vi "BuildCustomDashBoardData.vi"   [LabVIEW 2014]
doc: "This VI builds data and sends it back to the dashboard PC program. By default it sends back the raw values for the first analog, digital, and solenoid module. Modify it to send back the data you want to view. Consider adding higher level data to the Dashboard Datatype.ctl and to this VI. Then update the Dashboard to display the data however you like.\n\nThis software is licensed. Open the labview\\readme\\WPI Robotics Library Open Source License.txt file for more information."
uses:
  typedefs/test/test controls.ctl
  typedefs/fg_getset.ctl
  typedefs/dashboard/DashboardEnable.ctl
  <vilib>/Rock Robotics/SystemInterfaces/Typedef/FPGA_TypedefDigitalModule.ctl
  typedefs/dashboard/misc dash data.ctl
  <vilib>/Rock Robotics/WPI/Solenoid/WPI_SolenoidDevRef.ctl
  <vilib>/Rock Robotics/WPI/Solenoid/WPI_SolenoidChannel.ctl
  <vilib>/Rock Robotics/WPI/AnalogModule/WPI_AnalogModuleDevStatus.ctl
  <vilib>/Rock Robotics/SystemInterfaces/Typedef/FPGA_TypedefAnalogModule.ctl
  <vilib>/Rock Robotics/SystemInterfaces/AI/FPGA_AIChannel.ctl
  <vilib>/Rock Robotics/WPI/DriverStation/WPI_DriverStationDigitalData.ctl
  <vilib>/Rock Robotics/SystemInterfaces/DIO/FPGA_DIOPWMChannel.ctl
  <vilib>/Rock Robotics/WPI/Compressor/WPI_CompressorGetSetRefNum.vi
  <vilib>/Rock Robotics/Network Tables/SD Write Numeric Array.vi
  <vilib>/Rock Robotics/SystemInterfaces/System/FPGA_SystemGet.vi
  <vilib>/Rock Robotics/WPI/Solenoid/Deprecated/WPI_SolenoidGetBool.vi
  <vilib>/Rock Robotics/Network Tables/SD Write Boolean Array.vi
  <vilib>/NI_Real-Time Target Support.lvlib
panel:
  # "Generate Dashboard Data and Send it"
  # "Note: Test code calls some dashboard data, which is gotten there not here"
types:
  T1 = typedef "WPI_AnalogModuleDevStatus.ctl" = cluster{"DevStatus":errorcluster, "Controller":T2}
  T2 = typedef "FPGA_TypedefAnalogModule.ctl" = enum16{"Controller 1"}
  T3 = typedef "FPGA_AIChannel.ctl" = enum8{"AI 0", "AI 1", "AI 2", "AI 3", "AI MXP 0", "AI MXP 1", "AI MXP 2", "AI MXP 3", "Invalid"}
  T4 = typedef "FPGA_TypedefDigitalModule.ctl" = enum16{"Controller 1"}
  T5 = typedef "WPI_DriverStationDigitalData.ctl" = cluster{"Relay Fwd":u8, "Relay Rev":u8, "GPIO":u16, "GPIO_OE":u16, "PWM":cluster{"PWM[0]":u8, "PWM[1]":u8, "PWM[2]":u8, "PWM[3]":u8, "PWM[4]":u8, "PWM[5]":u8, "PWM[6]":u8, "PWM[7]":u8, "PWM[8]":u8, "PWM[9]":u8}}
  T6 = typedef "FPGA_DIOPWMChannel.ctl" = enum8{"PWM 0", "PWM 1", "PWM 2", "PWM 3", "PWM 4", "PWM 5", "PWM 6", "PWM 7", "PWM 8", "PWM 9", "PWM MXP 0", "PWM MXP 1", "PWM MXP 2", "PWM MXP 3", "PWM MXP 4", "PWM MXP 5", "PWM MXP 6", "PWM MXP 7", "PWM MXP 8", "PWM MXP 9", "Invalid"}
  T7 = typedef "WPI_SolenoidChannel.ctl" = enum8{"Solenoid 0", "Solenoid 1", "Solenoid 2", "Solenoid 3", "Solenoid 4", "Solenoid 5", "Solenoid 6", "Solenoid 7", "Invalid"}
  T8 = typedef "WPI_SolenoidDevRef.ctl" = cluster{"DevStatus":errorcluster, "Pneumatics Control Module":u8, "Forward Solenoid Channel":T7, "Reverse Solenoid Channel":T7}
  T9 = typedef "misc dash data.ctl" = cluster{"Total (%)":dbl, "Vision mSPI":u32, "Main mSPI":u32, "Vision":cluster{"distance":dbl}, "Enabled?":bool}
  T10 = typedef "DashboardEnable.ctl" = cluster{"Analog I/O":bool[], "Digital I/O":bool, "Solenoids":bool}
  T11 = typedef "subStates.ctl" = enum16{"null", "wait", "driver control", "auto", "manual override", "hold position", "rotate", "test", "end"}
  T12 = typedef "FPGA_DIODevRef.ctl" = cluster{"DevStatus":errorcluster, "Controller":T4}
  T13 = cluster{"[0]":u16, "[1]":u16, "[2]":u16, "[3]":u16, "[4]":u16, "[5]":u16, "[6]":u16, "[7]":u16, "[8]":u16, "[9]":u16}
  T14 = typedef "WPI_EncoderDevRef.ctl" = cluster{"DevStatus":errorcluster, "EncoderIndex":T15, "CounterIndex":T16, "DistancePerCount":dbl, "Decoding Type":T17}
  T15 = typedef "FPGA_EncoderIdx.ctl" = enum8{"Enc 0", "Enc 1", "Enc 2", "Enc 3", "Enc 4", "Enc 5", "Enc 6", "Enc 7", "Invalid"}
  T16 = typedef "FPGA_CounterCtrSystemIndex.ctl" = enum8{"Ctr 0", "Ctr 1", "Ctr 2", "Ctr 3", "Ctr 4", "Ctr 5", "Ctr 6", "Ctr 7", "Invalid"}
  T17 = typedef "WPI_EncoderType.ctl" = enum16{"1x", "2x", "4x"}
  T18 = typedef "WPI_CompressorDevRef.ctl" = cluster{"DevStatus":errorcluster, "Pneumatics Control Module":u8}
  T19 = typedef "fg_getset.ctl" = enum16{"Get", "Set"}
  T20 = typedef "NI_Real-Time Target Support.lvlib/RT CPU Load.ctl" = cluster{"Total (%)":dbl, "Time Critical (%)":dbl, "Timed Structures (%)":dbl, "High (%)":dbl, "Above Normal (%)":dbl, "Normal (%)":dbl, "Background (%)":dbl, "Idle (%)":dbl, "ISR (%)":dbl}
  T21 = cluster{"Vision mSPI":u32, "Main mSPI":u32, "Dash mSPI":u32}
  T22 = typedef "test controls.ctl" = cluster{"Button":bool, "Switch":bool, "Slider":dbl}
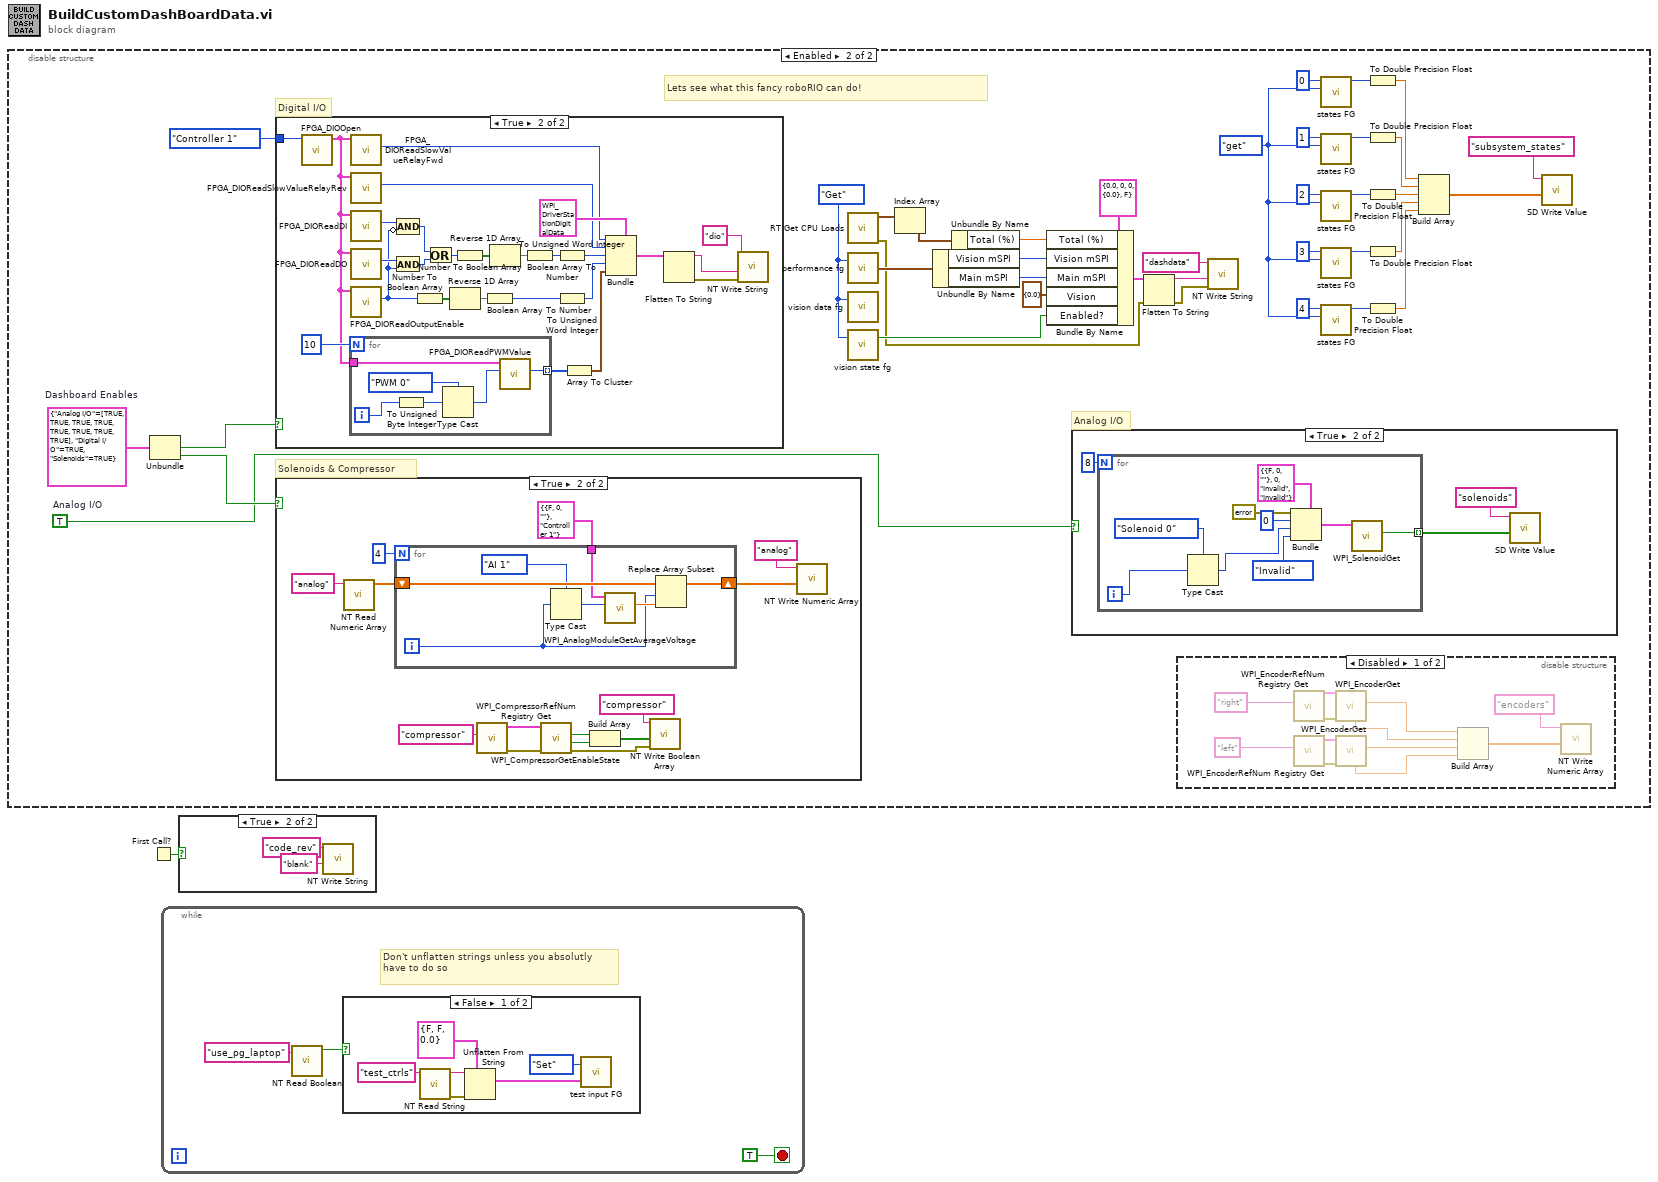
[diagram p0: block diagram]
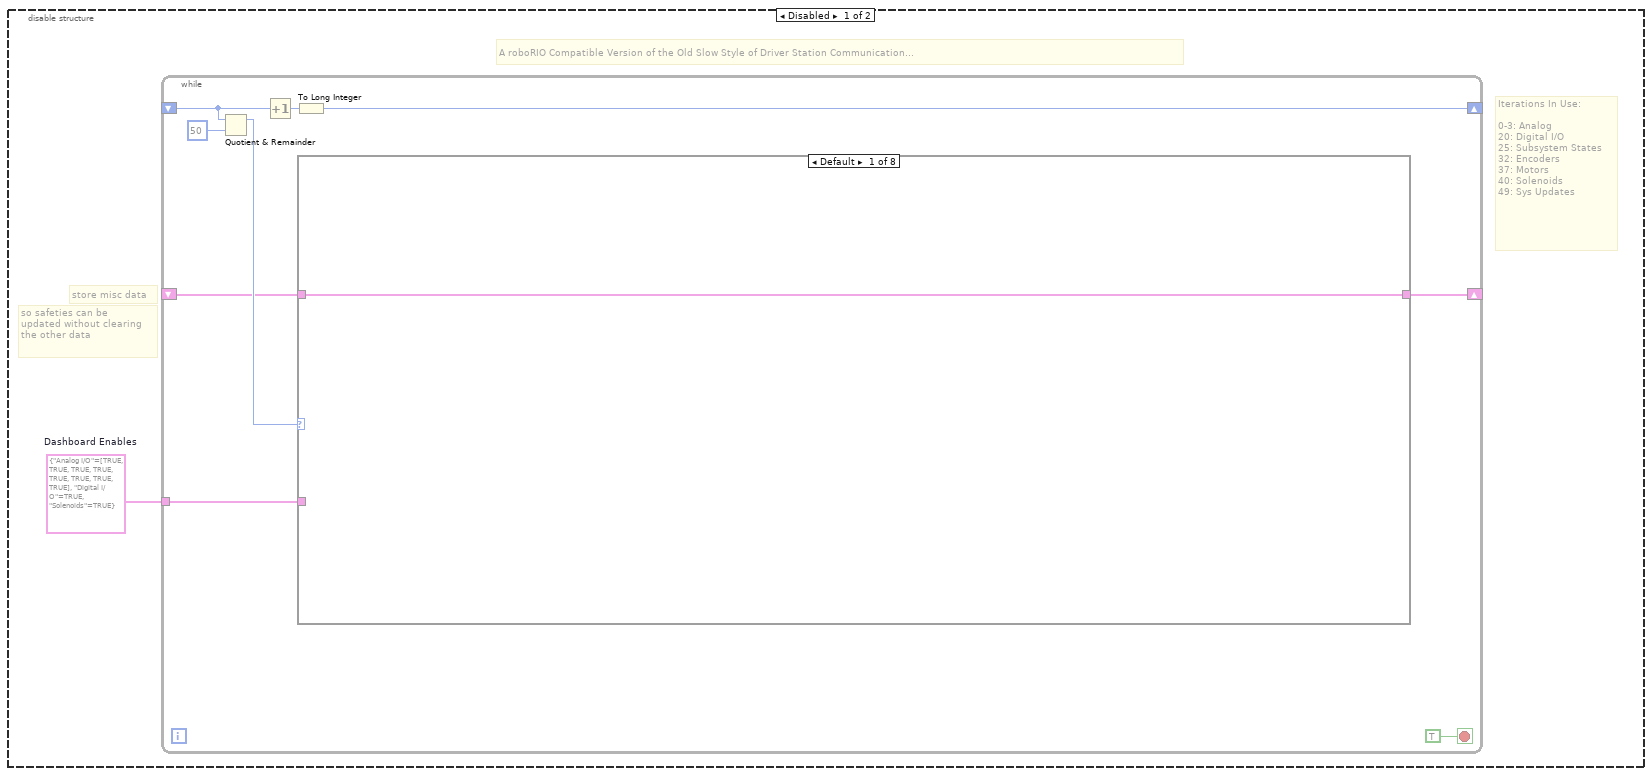
[diagram p2: hidden frame]
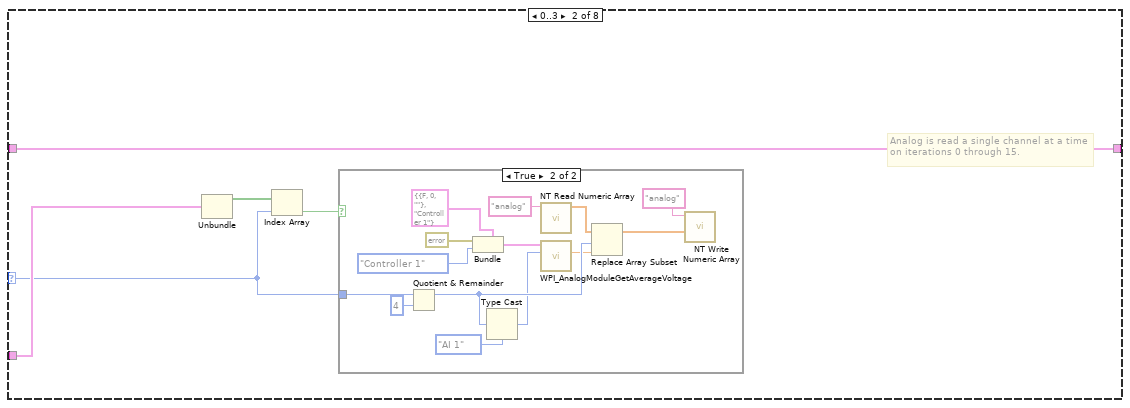
[diagram p3: hidden frame]
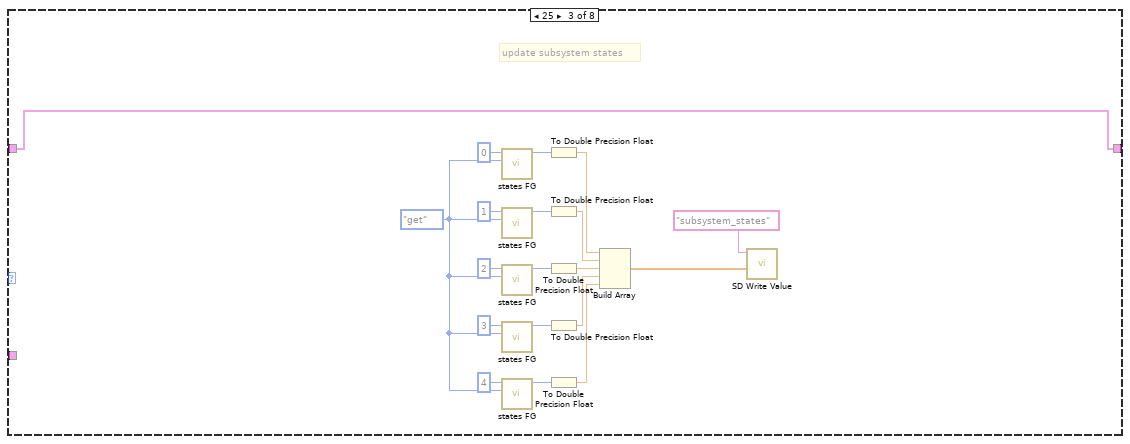
[diagram p5: hidden frame]
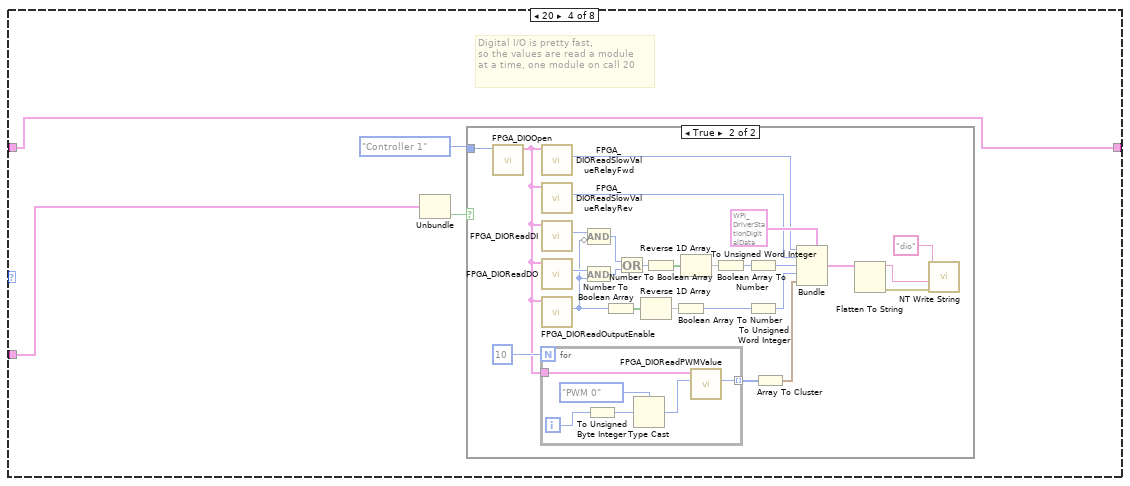
[diagram p6: hidden frame]
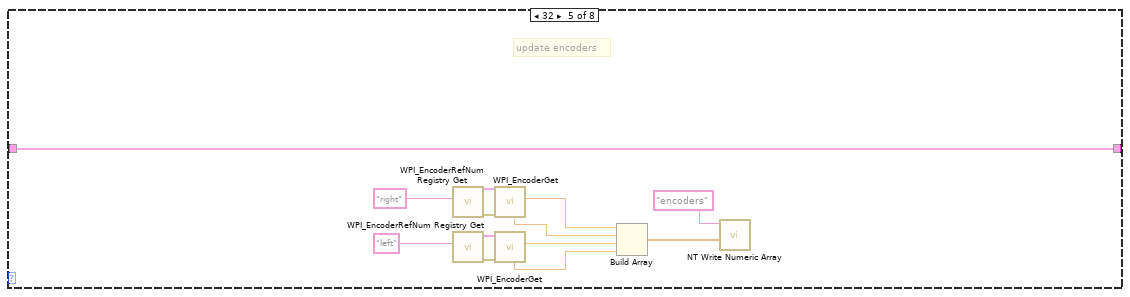
[diagram p8: hidden frame]
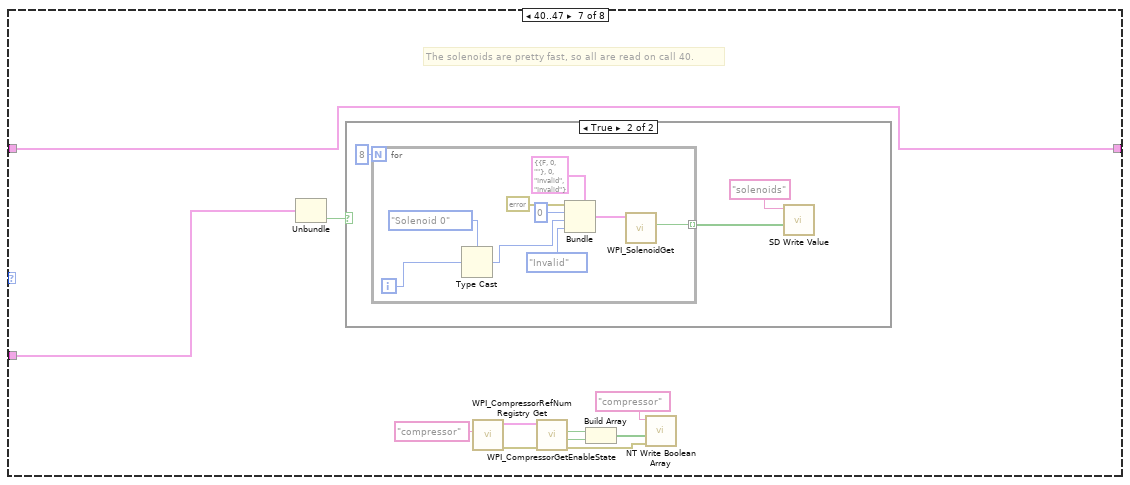
[diagram p10: hidden frame]
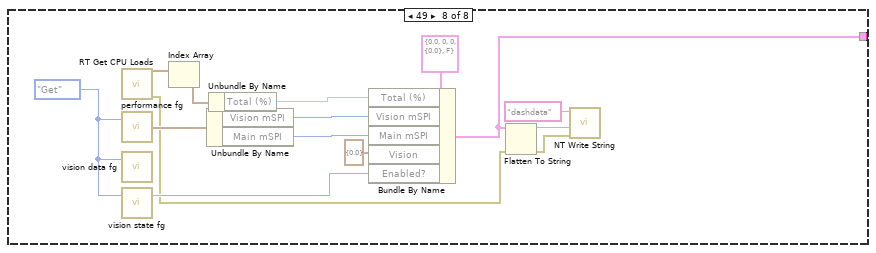
[diagram p12: hidden frame]
diagram:
  n1 = disable-structure shown="Enabled" {
    frame Disabled {
      w2 = T10 {"Analog I/O"=[TRUE, TRUE, TRUE, TRUE, TRUE, TRUE, TRUE, TRUE], "Digital I/O"=TRUE, "Solenoids"=TRUE}  # Dashboard Enables
      # "A roboRIO Compatible Version of the Old Slow Style of Driver Station Communication..."
      # "so safeties can be\nupdated without clearing\nthe other data"
      # "store misc data"
      # "Iterations In Use:\n\n0-3: Analog\n20: Digital I/O \n25: Subsystem States\n32: Encoders\n37: Motors\n40: Solenoids\n49: Sys Updates"
      n2 = while {
        shift-right: [w8] -> _
        shift-left: _ -> [w9]
        tunnel: w2 -> [w6]
        shift-right: [w4] -> _
        shift-left: _ -> [w3]
        stop <- TRUE stop-if-true
        n3 = Quotient & Remainder(x=w9, y=50) -> (x-y*floor(x/y)=w5:i32)  [unwired: 1 out]
        n4 = Increment(x=w9) -> (x+1=w10:i32)
        n5 = To Long Integer(number=w10) -> (32bit integer=w8:i32)
        n6 = case shown="Default" w5 {
          selector: w5 -> [_ w16 _ _ _ _ _ _]
          tunnel: w6 -> [_ w17 _ w54 _ _ w111 _]
          tunnel: [w12 w14 w33 w51 w89 w100 w102 w125] -> w4
          tunnel: w3 -> [w12 w14 w33 w51 w89 w100 w102 _]
          frame Default {
          }
          frame 0..3 {
            # "Analog is read a single channel at a time\non iterations 0 through 15."
            n7 = Unbundle(w17) -> ("Analog I/O"=w13:bool[])  [unwired: 2 out]
            n8 = Index Array(array=w13, index=w16) -> (element=w15:bool)
            n9 = case shown="True" w15 {
              tunnel: w16 -> [_ w29]
              frame False {
              }
              frame True {
                n10 = Quotient & Remainder(x=w29, y=4) -> (x-y*floor(x/y)=w23:i32)  [unwired: 1 out]
                n11 = Bundle(cluster=T1 {"DevStatus"={"status"=FALSE, "code"=0, "source"=""}, "Controller"=enum."Controller 1"} ("AnalogModuleDevStatus"), "DevStatus"=errorcluster {"status"=FALSE, "code"=0, "source"=""}, "Controller"=FPGA_TypedefAnalogModule."Controller 1") -> (w20:T1)
                n12 = Type Cast(type=FPGA_AIChannel."AI 1" ("Channel"), x=w23) -> (*(type *) &x=w22:T3)
                n13 = call <vilib>:"NT Read Numeric Array.vi"("Name"="analog") -> ("Numeric Array"=w27:dbl[])  [unwired: 9 in, 1 out]
                n14 = call <vilib>:"WPI_AnalogModuleGetAverageVoltage.vi"("Channel"=w22, "AnalogModuleDevStatus"=w20) -> ("Average Voltage"=w18:dbl)  [unwired: 1 in, 8 out]
                n15 = Replace Array Subset(array=w27, new element=w18, index=w23) -> (w25:dbl[])
                n16 = call <vilib>:"NT Write Numeric Array.vi"("Numeric Array"=w25, "Name"="analog") -> ()  [unwired: 9 in, 1 out]
              }
            }
          }
          frame 25 {
            w45 = enum16{"set", "get"}."get" ("menu (get)")
            # "update subsystem states"
            n17 = call "states FG.vi"("menu (get)"=w45, "Loop ID"=0) -> ("subState out"=w42:T11)  [unwired: 6 in, 3 out]
            n18 = call "states FG.vi"("menu (get)"=w45, "Loop ID"=1) -> ("subState out"=w43:T11)  [unwired: 6 in, 3 out]
            n19 = call "states FG.vi"("menu (get)"=w45, "Loop ID"=2) -> ("subState out"=w44:T11)  [unwired: 6 in, 3 out]
            n20 = call "states FG.vi"("menu (get)"=w45, "Loop ID"=3) -> ("subState out"=w41:T11)  [unwired: 6 in, 3 out]
            n21 = call "states FG.vi"("menu (get)"=w45, "Loop ID"=4) -> ("subState out"=w40:T11)  [unwired: 6 in, 3 out]
            n22 = To Double Precision Float(number=w42) -> (double precision float=w38:dbl)
            n23 = To Double Precision Float(number=w43) -> (double precision float=w37:dbl)
            n24 = To Double Precision Float(number=w44) -> (double precision float=w36:dbl)
            n25 = To Double Precision Float(number=w41) -> (double precision float=w35:dbl)
            n26 = To Double Precision Float(number=w40) -> (double precision float=w34:dbl)
            n27 = Build Array(w38, w37, w36, w35, w34) -> (w32:dbl[])
            n28 = call-poly <vilib>:"SD Write Value.vi"("Numeric Array"=w32, "Name"="subsystem_states") -> ()  [unwired: 8 in, 2 out]
          }
          frame 20 {
            # "Digital I/O is pretty fast,\nso the values are read a module\nat a time, one module on call 20"
            n29 = Unbundle(w54) -> ("Solenoids"=w52:bool)  [unwired: 2 out]
            n30 = case shown="True" w52 {
              tunnel: FPGA_TypedefDigitalModule."Controller 1" ("Module (Module 1)") -> [_ w61]
              frame False {
              }
              frame True {
                n31 = call <vilib>:"FPGA_DIOOpen.vi"("Controller"=w61) -> ("DIODeviceRef"=w77:T12)  [unwired: 1 in, 9 out]
                n32 = for {
                  N: 10 -> [_]
                  tunnel: w77 -> [w86]
                  tunnel: [w84] -> w78 mode=indexing
                  i -> [w85]
                  n33 = To Unsigned Byte Integer(number=w85) -> (unsigned 8bit integer=w83:u8)
                  n34 = Type Cast(type=FPGA_DIOPWMChannel."PWM 0" ("PWMChannel"), x=w83) -> (*(type *) &x=w81:T6)
                  n35 = call <vilib>:"FPGA_DIOReadPWMValue.vi"("PWMChannel"=w81, "DIODeviceRef In"=w86) -> ("PWMValue"=w84:u16)  [unwired: 1 in, 8 out]
                }
                n36 = call <vilib>:"FPGA_DIOReadSlowValueRelayFwd.vi"("DIODeviceRef In"=w77) -> ("Relay Forward"=w70:u8)  [unwired: 1 in, 9 out]
                n37 = call <vilib>:"FPGA_DIOReadSlowValueRelayRev.vi"("DIODeviceRef In"=w77) -> ("Relay Reverse"=w71:u8)  [unwired: 1 in, 9 out]
                n38 = call <vilib>:"FPGA_DIOReadDI.vi"("DIODeviceRef In"=w77) -> ("DI"=w75:u32)  [unwired: 1 in, 9 out]
                n39 = call <vilib>:"FPGA_DIOReadDO.vi"("DIODeviceRef In"=w77) -> ("DO"=w74:u32)  [unwired: 1 in, 9 out]
                n40 = call <vilib>:"FPGA_DIOReadOutputEnable.vi"("DIODeviceRef In"=w77) -> ("OutputEnable"=w65:u32)  [unwired: 1 in, 9 out]
                n41 = And(x=w74, y=w65) -> (x .and. y?=w73:u32)
                n42 = Compound Arithmetic op=AND(w75, invert w65) -> (w72:u32)
                n43 = Number To Boolean Array(number=w65) -> (Boolean array=w67:bool[])
                n44 = Or(x=w72, y=w73) -> (x .or. y?=w63:u32)
                n45 = Reverse 1D Array(array=w67) -> (reversed array=w66:bool[])
                n46 = Number To Boolean Array(number=w63) -> (Boolean array=w68:bool[])
                n47 = Boolean Array To Number(Boolean array=w66) -> (number=w64:u32)
                n48 = Reverse 1D Array(array=w68) -> (reversed array=w69:bool[])
                n49 = Boolean Array To Number(Boolean array=w69) -> (number=w62:u32)
                n50 = To Unsigned Word Integer(number=w62) -> (unsigned 16bit integer=w55:u16)
                n51 = To Unsigned Word Integer(number=w64) -> (unsigned 16bit integer=w56:u16)
                n52 = Array To Cluster(array=w78) -> (cluster=w76:T13)
                n53 = Bundle(cluster=T5 {"Relay Fwd"=0, "Relay Rev"=0, "GPIO"=0, "GPIO_OE"=0, "PWM"={"PWM[0]"=0, "PWM[1]"=0, "PWM[2]"=0, "PWM[3]"=0, "PWM[4]"=0, "PWM[5]"=0, "PWM[6]"=0, "PWM[7]"=0, "PWM[8]"=0, "PWM[9]"=0}} ("DigitalModule"), "Relay Fwd"=w70, "Relay Rev"=w71, "GPIO"=w55, "GPIO_OE"=w56, "PWM"=w76) -> (w60:T5)
                n54 = Flatten To String(anything=w60) -> (data string=w58:string, error out=w59:errorcluster)  [unwired: 1 in, 3 out]
                n55 = call <vilib>:"NT Write String.vi"("error in"=w59, "String"=w58, "Name"="dio") -> ()  [unwired: 8 in, 1 out]
              }
            }
          }
          frame 32 {
            # "update encoders"
            n56 = call <vilib>:"WPI_EncoderRefNum Registry Get.vi"("refnum name"="right") -> ("error out"=w97:errorcluster, "EncoderDevRef"=w96:T14)  [unwired: 9 in]
            n57 = call <vilib>:"WPI_EncoderRefNum Registry Get.vi"("refnum name"="left") -> ("error out"=w94:errorcluster, "EncoderDevRef"=w95:T14)  [unwired: 9 in]
            n58 = call <vilib>:"WPI_EncoderGet.vi"("error in (no error)"=w97, "EncoderDevRef"=w96) -> ("Distance"=w93:dbl, "Rate"=w88:dbl)  [unwired: 4 in, 4 out]
            n59 = call <vilib>:"WPI_EncoderGet.vi"("error in (no error)"=w94, "EncoderDevRef"=w95) -> ("Distance"=w92:dbl, "Rate"=w91:dbl)  [unwired: 4 in, 4 out]
            n60 = Build Array(w93, w88, w92, w91) -> (w90:dbl[])
            n61 = call <vilib>:"NT Write Numeric Array.vi"("Numeric Array"=w90, "Name"="encoders") -> ()  [unwired: 9 in, 1 out]
          }
          frame 37 {
            # "update motor array"
          }
          frame 40..47 {
            # "The solenoids are pretty fast, so all are read on call 40."
            n62 = Unbundle(w111) -> ("Solenoids"=w101:bool)  [unwired: 2 out]
            n63 = case shown="True" w101 {
              frame False {
              }
              frame True {
                n64 = for {
                  N: 8 -> [_]
                  tunnel: [w115] -> w113 mode=indexing
                  i -> [w117]
                  n65 = Type Cast(type=WPI_SolenoidChannel."Solenoid 0" ("Forward Solenoid Channel"), x=w117) -> (*(type *) &x=w116:T7)
                  n66 = Bundle(cluster=T8 {"DevStatus"={"status"=FALSE, "code"=0, "source"=""}, "Pneumatics Control Module"=0, "Forward Solenoid Channel"=enum."Invalid", "Reverse Solenoid Channel"=enum."Invalid"} ("SolenoidDevRef"), "DevStatus"=errorcluster {"status"=FALSE, "code"=0, "source"=""}, "Pneumatics Control Module"=u8 0, "Forward Solenoid Channel"=w116, "Reverse Solenoid Channel"=WPI_SolenoidChannel."Invalid") -> (w122:T8)
                  n67 = call-poly <vilib>:"WPI_SolenoidGet.vi"("SolenoidDevRef"=w122) -> ("Value"=w115:bool)  [unwired: 8 in, 2 out]
                }
                n68 = call-poly <vilib>:"SD Write Value.vi"("Boolean Array"=w113, "Name"="solenoids") -> ()  [unwired: 8 in, 2 out]
              }
            }
            n69 = call <vilib>:"WPI_CompressorRefNum Registry Get.vi"("refnum name"="compressor") -> ("error out"=w107:errorcluster, "CompressorDevRef"=w108:T18)  [unwired: 9 in]
            n70 = call <vilib>:"WPI_CompressorGetEnableState.vi"("error in (no error)"=w107, "CompressorDevRef"=w108) -> ("error out"=w103:errorcluster, "Compressor Running"=w105:bool, "Enabled"=w106:bool)  [unwired: 6 in, 1 out]
            n71 = Build Array(w106, w105) -> (w104:bool[])
            n72 = call <vilib>:"NT Write Boolean Array.vi"("error in"=w103, "Boolean Array"=w104, "Name"="compressor") -> ()  [unwired: 8 in, 1 out]
          }
          frame 49 {
            w135 = fg_getset."Get" ("Menu")
            n73 = call <vilib>:"RT Get CPU Loads.vi"() -> ("error out"=w126:errorcluster, "CPU loads"=w137:T20[])  [unwired: 10 in]
            n74 = call "performance fg.vi"("Menu"=w135) -> ("Output"=w136:T21)  [unwired: 1 in]
            n75 = call "vision data fg.vi"("Menu"=w135) -> ()  [unwired: 1 in, 1 out]
            n76 = call "vision state fg.vi"("Menu"=w135) -> ("Enabled?"=w133:bool)  [unwired: 1 in, 1 out]
            n77 = Index Array(array=w137) -> (element=w138:T20)  [unwired: 1 in]
            n78 = Unbundle By Name(w136) -> ("Vision mSPI"=w131:u32, "Main mSPI"=w132:u32)
            n79 = Unbundle By Name(w138) -> ("Total (%)"=w130:dbl)
            n80 = Bundle By Name(cluster=T9 {"Total (%)"=0.0, "Vision mSPI"=0, "Main mSPI"=0, "Vision"={"distance"=0.0}, "Enabled?"=FALSE}, "Total (%)"=w130, "Vision mSPI"=w131, "Main mSPI"=w132, "Vision"=cluster{"distance":dbl} {"distance"=0.0}, "Enabled?"=w133) -> (w125:T9)
            n81 = Flatten To String(anything=w125, error in (no error)=w126) -> (data string=w129:string, error out=w127:errorcluster)  [unwired: 3 out]
            n82 = call <vilib>:"NT Write String.vi"("error in"=w127, "String"=w129, "Name"="dashdata") -> ()  [unwired: 8 in, 1 out]
          }
        }
      }
    }
    frame Enabled {
      w150 = fg_getset."Get" ("Menu")
      w154 = TRUE  # Analog I/O
      w169 = enum16{"set", "get"}."get" ("menu (get)")
      w176 = T10 {"Analog I/O"=[TRUE, TRUE, TRUE, TRUE, TRUE, TRUE, TRUE, TRUE], "Digital I/O"=TRUE, "Solenoids"=TRUE}  # Dashboard Enables
      # "Analog I/O"
      # "Digital I/O"
      # "Solenoids & Compressor"
      # "Lets see what this fancy roboRIO can do!"
      n83 = Unbundle(w176) -> ("Digital I/O"=w155:bool, "Solenoids"=w175:bool)  [unwired: 1 out]
      n84 = case shown="True" w155 {
        tunnel: FPGA_TypedefDigitalModule."Controller 1" ("Module (Module 1)") -> [_ w195]
        frame False {
        }
        frame True {
          n85 = call <vilib>:"FPGA_DIOOpen.vi"("Controller"=w195) -> ("DIODeviceRef"=w211:T12)  [unwired: 1 in, 9 out]
          n86 = for {
            N: 10 -> [_]
            tunnel: w211 -> [w220]
            tunnel: [w218] -> w212 mode=indexing
            i -> [w219]
            n87 = To Unsigned Byte Integer(number=w219) -> (unsigned 8bit integer=w217:u8)
            n88 = Type Cast(type=FPGA_DIOPWMChannel."PWM 0" ("PWMChannel"), x=w217) -> (*(type *) &x=w215:T6)
            n89 = call <vilib>:"FPGA_DIOReadPWMValue.vi"("PWMChannel"=w215, "DIODeviceRef In"=w220) -> ("PWMValue"=w218:u16)  [unwired: 1 in, 8 out]
          }
          n90 = call <vilib>:"FPGA_DIOReadSlowValueRelayFwd.vi"("DIODeviceRef In"=w211) -> ("Relay Forward"=w204:u8)  [unwired: 1 in, 9 out]
          n91 = call <vilib>:"FPGA_DIOReadSlowValueRelayRev.vi"("DIODeviceRef In"=w211) -> ("Relay Reverse"=w205:u8)  [unwired: 1 in, 9 out]
          n92 = call <vilib>:"FPGA_DIOReadDI.vi"("DIODeviceRef In"=w211) -> ("DI"=w209:u32)  [unwired: 1 in, 9 out]
          n93 = call <vilib>:"FPGA_DIOReadDO.vi"("DIODeviceRef In"=w211) -> ("DO"=w208:u32)  [unwired: 1 in, 9 out]
          n94 = call <vilib>:"FPGA_DIOReadOutputEnable.vi"("DIODeviceRef In"=w211) -> ("OutputEnable"=w199:u32)  [unwired: 1 in, 9 out]
          n95 = And(x=w208, y=w199) -> (x .and. y?=w207:u32)
          n96 = Compound Arithmetic op=AND(w209, invert w199) -> (w206:u32)
          n97 = Number To Boolean Array(number=w199) -> (Boolean array=w201:bool[])
          n98 = Or(x=w206, y=w207) -> (x .or. y?=w197:u32)
          n99 = Reverse 1D Array(array=w201) -> (reversed array=w200:bool[])
          n100 = Number To Boolean Array(number=w197) -> (Boolean array=w202:bool[])
          n101 = Boolean Array To Number(Boolean array=w200) -> (number=w198:u32)
          n102 = Reverse 1D Array(array=w202) -> (reversed array=w203:bool[])
          n103 = Boolean Array To Number(Boolean array=w203) -> (number=w196:u32)
          n104 = To Unsigned Word Integer(number=w196) -> (unsigned 16bit integer=w189:u16)
          n105 = To Unsigned Word Integer(number=w198) -> (unsigned 16bit integer=w190:u16)
          n106 = Array To Cluster(array=w212) -> (cluster=w210:T13)
          n107 = Bundle(cluster=T5 {"Relay Fwd"=0, "Relay Rev"=0, "GPIO"=0, "GPIO_OE"=0, "PWM"={"PWM[0]"=0, "PWM[1]"=0, "PWM[2]"=0, "PWM[3]"=0, "PWM[4]"=0, "PWM[5]"=0, "PWM[6]"=0, "PWM[7]"=0, "PWM[8]"=0, "PWM[9]"=0}} ("DigitalModule"), "Relay Fwd"=w204, "Relay Rev"=w205, "GPIO"=w189, "GPIO_OE"=w190, "PWM"=w210) -> (w194:T5)
          n108 = Flatten To String(anything=w194) -> (data string=w192:string, error out=w193:errorcluster)  [unwired: 1 in, 3 out]
          n109 = call <vilib>:"NT Write String.vi"("error in"=w193, "String"=w192, "Name"="dio") -> ()  [unwired: 8 in, 1 out]
        }
      }
      n110 = case shown="True" w175 {
        frame False {
        }
        frame True {
          n111 = call <vilib>:"NT Read Numeric Array.vi"("Name"="analog") -> ("Numeric Array"=w237:dbl[])  [unwired: 9 in, 1 out]
          n112 = for {
            N: 4 -> [_]
            tunnel: T1 {"DevStatus"={"status"=FALSE, "code"=0, "source"=""}, "Controller"=enum."Controller 1"} ("AnalogModuleDevStatus") -> [w248]
            shift-right: [w252] -> w236
            shift-left: w237 -> [w253]
            i -> [w247]
            n113 = Type Cast(type=FPGA_AIChannel."AI 1" ("Channel"), x=w247) -> (*(type *) &x=w250:T3)
            n114 = call <vilib>:"WPI_AnalogModuleGetAverageVoltage.vi"("Channel"=w250, "AnalogModuleDevStatus"=w248) -> ("Average Voltage"=w249:dbl)  [unwired: 1 in, 8 out]
            n115 = Replace Array Subset(array=w253, new element=w249, index=w247) -> (w252:dbl[])
          }
          n116 = call <vilib>:"WPI_CompressorRefNum Registry Get.vi"("refnum name"="compressor") -> ("error out"=w243:errorcluster, "CompressorDevRef"=w244:T18)  [unwired: 9 in]
          n117 = call <vilib>:"WPI_CompressorGetEnableState.vi"("error in (no error)"=w243, "CompressorDevRef"=w244) -> ("error out"=w239:errorcluster, "Compressor Running"=w241:bool, "Enabled"=w242:bool)  [unwired: 6 in, 1 out]
          n118 = Build Array(w242, w241) -> (w240:bool[])
          n119 = call <vilib>:"NT Write Boolean Array.vi"("error in"=w239, "Boolean Array"=w240, "Name"="compressor") -> ()  [unwired: 8 in, 1 out]
          n120 = call <vilib>:"NT Write Numeric Array.vi"("Numeric Array"=w236, "Name"="analog") -> ()  [unwired: 9 in, 1 out]
        }
      }
      n121 = call <vilib>:"RT Get CPU Loads.vi"() -> ("error out"=w141:errorcluster, "CPU loads"=w152:T20[])  [unwired: 10 in]
      n122 = call "performance fg.vi"("Menu"=w150) -> ("Output"=w151:T21)  [unwired: 1 in]
      n123 = call "vision data fg.vi"("Menu"=w150) -> ()  [unwired: 1 in, 1 out]
      n124 = call "vision state fg.vi"("Menu"=w150) -> ("Enabled?"=w148:bool)  [unwired: 1 in, 1 out]
      n125 = Index Array(array=w152) -> (element=w153:T20)  [unwired: 1 in]
      n126 = Unbundle By Name(w151) -> ("Vision mSPI"=w146:u32, "Main mSPI"=w147:u32)
      n127 = Unbundle By Name(w153) -> ("Total (%)"=w145:dbl)
      n128 = Bundle By Name(cluster=T9 {"Total (%)"=0.0, "Vision mSPI"=0, "Main mSPI"=0, "Vision"={"distance"=0.0}, "Enabled?"=FALSE}, "Total (%)"=w145, "Vision mSPI"=w146, "Main mSPI"=w147, "Vision"=cluster{"distance":dbl} {"distance"=0.0}, "Enabled?"=w148) -> (w140:T9)
      n129 = case shown="True" w154 {
        frame False {
        }
        frame True {
          n130 = for {
            N: 8 -> [_]
            tunnel: [w180] -> w178 mode=indexing
            i -> [w182]
            n131 = Type Cast(type=WPI_SolenoidChannel."Solenoid 0" ("Forward Solenoid Channel"), x=w182) -> (*(type *) &x=w181:T7)
            n132 = Bundle(cluster=T8 {"DevStatus"={"status"=FALSE, "code"=0, "source"=""}, "Pneumatics Control Module"=0, "Forward Solenoid Channel"=enum."Invalid", "Reverse Solenoid Channel"=enum."Invalid"} ("SolenoidDevRef"), "DevStatus"=errorcluster {"status"=FALSE, "code"=0, "source"=""}, "Pneumatics Control Module"=u8 0, "Forward Solenoid Channel"=w181, "Reverse Solenoid Channel"=WPI_SolenoidChannel."Invalid") -> (w187:T8)
            n133 = call-poly <vilib>:"WPI_SolenoidGet.vi"("SolenoidDevRef"=w187) -> ("Value"=w180:bool)  [unwired: 8 in, 2 out]
          }
          n134 = call-poly <vilib>:"SD Write Value.vi"("Boolean Array"=w178, "Name"="solenoids") -> ()  [unwired: 8 in, 2 out]
        }
      }
      n135 = Flatten To String(anything=w140, error in (no error)=w141) -> (data string=w144:string, error out=w142:errorcluster)  [unwired: 3 out]
      n136 = disable-structure shown="Disabled" {
        frame Disabled {
          n137 = call <vilib>:"WPI_EncoderRefNum Registry Get.vi"("refnum name"="right") -> ("error out"=w230:errorcluster, "EncoderDevRef"=w229:T14)  [unwired: 9 in]
          n138 = call <vilib>:"WPI_EncoderRefNum Registry Get.vi"("refnum name"="left") -> ("error out"=w227:errorcluster, "EncoderDevRef"=w228:T14)  [unwired: 9 in]
          n139 = call <vilib>:"WPI_EncoderGet.vi"("error in (no error)"=w230, "EncoderDevRef"=w229) -> ("Distance"=w226:dbl, "Rate"=w222:dbl)  [unwired: 4 in, 4 out]
          n140 = call <vilib>:"WPI_EncoderGet.vi"("error in (no error)"=w227, "EncoderDevRef"=w228) -> ("Distance"=w225:dbl, "Rate"=w224:dbl)  [unwired: 4 in, 4 out]
          n141 = Build Array(w226, w222, w225, w224) -> (w223:dbl[])
          n142 = call <vilib>:"NT Write Numeric Array.vi"("Numeric Array"=w223, "Name"="encoders") -> ()  [unwired: 9 in, 1 out]
        }
        frame Enabled {
        }
      }
      n143 = call <vilib>:"NT Write String.vi"("error in"=w142, "String"=w144, "Name"="dashdata") -> ()  [unwired: 8 in, 1 out]
      n144 = call "states FG.vi"("menu (get)"=w169, "Loop ID"=0) -> ("subState out"=w166:T11)  [unwired: 6 in, 3 out]
      n145 = call "states FG.vi"("menu (get)"=w169, "Loop ID"=1) -> ("subState out"=w167:T11)  [unwired: 6 in, 3 out]
      n146 = call "states FG.vi"("menu (get)"=w169, "Loop ID"=2) -> ("subState out"=w168:T11)  [unwired: 6 in, 3 out]
      n147 = call "states FG.vi"("menu (get)"=w169, "Loop ID"=3) -> ("subState out"=w165:T11)  [unwired: 6 in, 3 out]
      n148 = call "states FG.vi"("menu (get)"=w169, "Loop ID"=4) -> ("subState out"=w164:T11)  [unwired: 6 in, 3 out]
      n149 = To Double Precision Float(number=w166) -> (double precision float=w162:dbl)
      n150 = To Double Precision Float(number=w167) -> (double precision float=w161:dbl)
      n151 = To Double Precision Float(number=w168) -> (double precision float=w160:dbl)
      n152 = To Double Precision Float(number=w165) -> (double precision float=w159:dbl)
      n153 = To Double Precision Float(number=w164) -> (double precision float=w158:dbl)
      n154 = Build Array(w162, w161, w160, w159, w158) -> (w157:dbl[])
      n155 = call-poly <vilib>:"SD Write Value.vi"("Numeric Array"=w157, "Name"="subsystem_states") -> ()  [unwired: 8 in, 2 out]
    }
  }
  n156 = First Call?() -> (First Call?: T/F=w1:bool)
  n157 = while {
    stop <- TRUE stop-if-true
    # "Don't unflatten strings unless you absolutly\nhave to do so"
    n158 = call <vilib>:"NT Read Boolean.vi"("Name"="use_pg_laptop") -> ("Boolean"=w255:bool)  [unwired: 9 in, 1 out]
    n159 = case shown="False" w255 {
      frame False {
        n160 = call <vilib>:"NT Read String.vi"("Name"="test_ctrls") -> ("error out"=w261:errorcluster, "String"=w260:string)  [unwired: 9 in]
        n161 = Unflatten From String(type=T22 {"Button"=FALSE, "Switch"=FALSE, "Slider"=0.0} ("Test Controls"), binary string=w260, error in (no error)=w261) -> (value=w258:T22)  [unwired: 2 in, 2 out]
        n162 = call "test input FG.vi"("Test Controls"=w258, "Menu"=fg_getset."Set") -> ()  [unwired: 1 out]
      }
      frame True {
      }
    }
  }
  n163 = case shown="True" w1 {
    frame False {
    }
    frame True {
      n164 = call <vilib>:"NT Write String.vi"("String"="blank", "Name"="code_rev") -> ()  [unwired: 9 in, 1 out]
    }
  }
